vi "Destroy Suite.vi"(8 "error in":errorcluster, 11 "Platano":refnum<class "Platano.CarayaTestSuite.lvclass">) -> (0 "error out":errorcluster, 3 "Test Suite Results":refnum<class "Test Result.lvclass">)   [LabVIEW 2021, in "Banana.Caraya.lvlib" / "Platano.CarayaTestSuite.lvclass"]
uses:
  Banana/Banana.lvclass/Banana.ctl
  DefineSuite/DefineSuite.lvclass/DefineSuite.ctl
  DefineSuite/Write Interactive.vi
  <vilib>/LabVIEW Open Source Project/Data Manipulation/Variant/Variant_SetName.vi
  <vilib>/LabVIEW Open Source Project/Data Manipulation/Variant/Variant_BuildClusterFromElementArray.vi
  Banana/Read Ephemerals.vi
  <vilib>/LabVIEW Open Source Project/Data Manipulation/Variant/Variant_EmptyCluster.vi
  DefineSuite/DefineSuite.lvclass
  C:/Repositories/LVOS/Bananas/lv-src/Bananas/BananaPeel/BananaPeel.lvclass
  <vilib>/LabVIEW Open Source Project/Data Manipulation/Variant/Variant_ListElements.vi
  <vilib>/LabVIEW Open Source Project/Data Manipulation/TypeDescriptor/TypeDescriptor_SetName.vi
  <vilib>/Utility/GetType.llb/TD_Create Cluster.vi
  DefineTest/DefineTest.lvclass
  Banana.Caraya/Platano.CarayaTestSuite/Platano.CarayaTestSuite.lvclass
  Banana.Caraya/Platano.CarayaTestSuite/Platano.CarayaTestSuite.lvclass/Platano.CarayaTestSuite.ctl
  Banana/Banana.lvclass
  Platano/Platano.lvclass
  Banana Core Actions -- enum.ctl
  <vilib>/addons/_JKI Toolkits/Caraya/classes/Test Suite/Test Suite.lvclass
  DestroySuite/DestroySuite.lvclass
  C:/Repositories/LVOS/Bananas/lv-src/Bananas/DestroySuite/DestroySuite.lvclass
  C:/Repositories/LVOS/Bananas/lv-src/Banana.Caraya/Platano.CarayaTestSuite/Platano.CarayaTestSuite.lvclass
  C:/Repositories/LVOS/Bananas/lv-src/Bananas/Platano/Platano.lvclass
  <vilib>/addons/_JKI Toolkits/Caraya/classes/Test Result/Test Result.lvclass
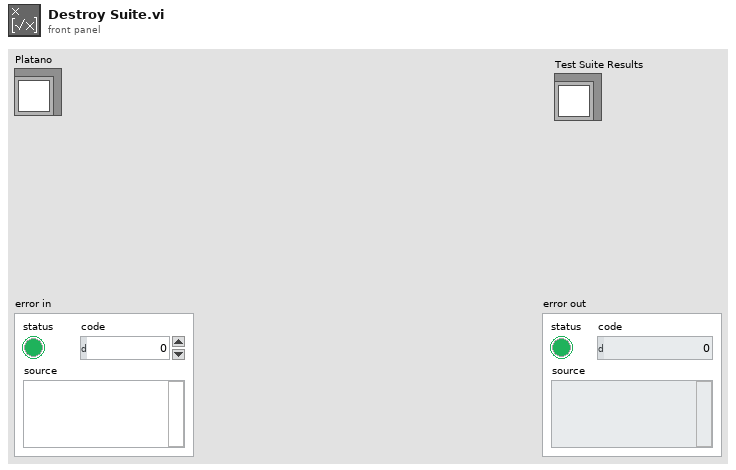
[diagram p1: front panel]
types:
  T1 = typedef "Bananas.lvlib/Test Strategies -- cluster.ctl" = cluster{"DefineTest":refnum<class "DefineTest.lvclass">, "DefineSuite":refnum<class "DefineSuite.lvclass">, "DestroySuite":refnum<class "DestroySuite.lvclass">}
  T2 = typedef "Bananas.lvlib/Platano.lvclass/Banana Core Actions -- enum.ctl" = enum16{"Get/Set", "Clear", "Discard"}
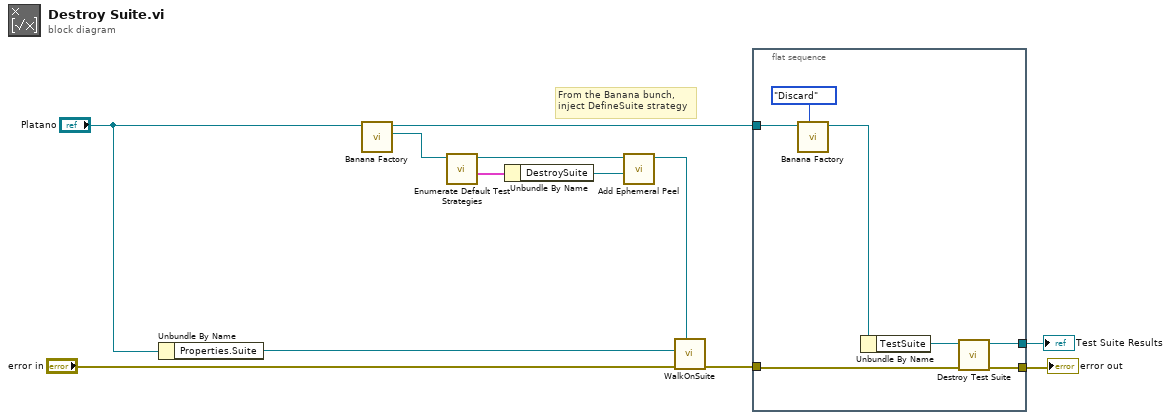
[diagram p0: block diagram]
diagram:
  # "From the Banana bunch,\ninject DefineSuite strategy"
  n1 = Unbundle By Name("Platano") -> ("Properties.Suite"=w9:refnum<class "Properties.Suite.lvclass">)
  n2 = call "Banana Factory.vi"("Platano"="Platano") -> ("Banana"=w7:refnum<class "Banana.lvclass">, "Platano dup"=w8:refnum<class "Platano.CarayaTestSuite.lvclass">)  [unwired: 9 in]
  n3 = call "Enumerate Default Test Strategies.vi"("Banana"=w7) -> ("Strategies"=w12:T1, "Banana"=w11:refnum<class "Banana.lvclass">)  [unwired: 9 in]
  n4 = Unbundle By Name(w12) -> ("DestroySuite"=w1:refnum<class "DestroySuite.lvclass">)
  n5 = call "Add Ephemeral Peel.vi"("BananaPeel"=w1, "Banana"=w11) -> ("Banana"=w10:refnum<class "Banana.lvclass">)  [unwired: 9 in]
  n6 = call "WalkOnSuite.vi"("Banana"=w10, "error in (no error)"="error in", "Properties.Suite"=w9) -> ("error out"=w3:errorcluster)  [unwired: 7 in, 1 out]
  n7 = flat-sequence {
    tunnel: w8 -> [w18]
    tunnel: w3 -> [w16]
    tunnel: [w17] -> w4
    tunnel: [w15] -> w2
    frame #0 {
      n8 = call "Banana Factory.vi"("Action"=Banana_Core_Actions_--_enum."Discard", "Platano"=w18) -> ("Platano dup"=w14:refnum<class "Platano.CarayaTestSuite.lvclass">)  [unwired: 8 in, 1 out]
      n9 = Unbundle By Name(w14) -> ("TestSuite"=w13:refnum<class "Test Suite.lvclass">)
      n10 = call-dynamic "Destroy Test Suite.vi"("error in (no error)"=w16, "Test Suite in"=w13) -> ("error out"=w15:errorcluster, "Test Suite Results"=w17:refnum<class "Test Result.lvclass">)  [unwired: 8 in]
    }
  }
  "error out" <- w2
  "Test Suite Results" <- w4
